vi "Get Endpoints from Switches JSON.vi"(8 "error in (no error)":errorcluster, 10 "topology":string, 11 "switches json":string) -> (0 "error out":errorcluster, 3 "endpoints":string[](array[string]))   [LabVIEW 2017, in "SLSC Switch Scripting.lvlib"]
uses:
  SLSC Switch Scripting.lvlib
  <vilib>/SLSC_Switch/Initialize with Topology (Simulate).vi
  <vilib>/SLSC_Switch/SLSC Switch.lvlib
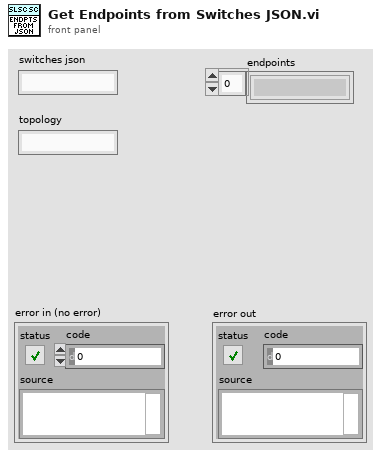
[diagram p1: front panel]
types:
  T1 = typedef "nislscslSession.ctl" = refnum<k20>
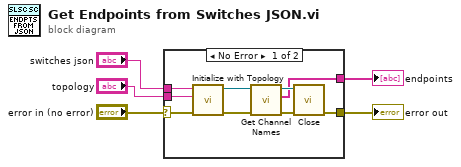
[diagram p0: block diagram]
diagram:
  n1 = case shown="No Error" "error in (no error)" {
    selector: "error in (no error)" -> [w14 w15]
    tunnel: "switches json" -> [w13 _]
    tunnel: "topology" -> [w12 _]
    tunnel: [w7 _] -> w2
    tunnel: [w6 w15] -> w1
    frame No Error {
      n2 = call-poly <vilib>:"Initialize with Topology.vi"("error in (no error)"=w14, "topology"=w12, "switches json"=w13) -> ("error out"=w10:errorcluster, "session out"=w11:T1)  [unwired: 7 in]
      n3 = call <vilib>:"Get Channel Names.vi"("error in (no error)"=w10, "session in"=w11) -> ("error out"=w8:errorcluster, "channel names"=w7:string[], "session out"=w9:T1)  [unwired: 7 in]
      n4 = call <vilib>:"Close.vi"("error in (no error)"=w8, "session in"=w9) -> ("error out"=w6:errorcluster)  [unwired: 9 in]
    }
    frame Error {
    }
  }
  "error out" <- w1
  "endpoints" <- w2
